vi "RichToFlatrfcontrol_DeviceStatusResponse.vi"(5 "OutputClusterType":T1, 11 "InputCluster":T2) -> (3 "OutputCluster":T1)   [LabVIEW 2024, in "FlexSDR_gRPC_client.lvlib"]
uses:
  rfcontrol_DeviceStatusResponse.ctl
  rfcontrol_DeviceStatusResponse_Flat.ctl
  FlexSDR_gRPC_client.lvlib
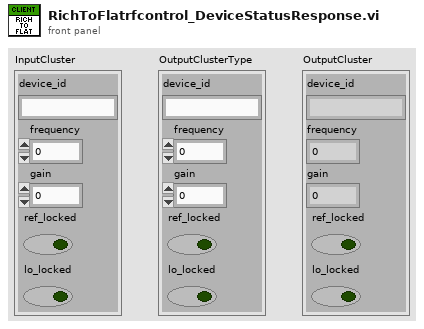
[diagram p1: front panel]
types:
  T1 = typedef "FlexSDR_gRPC_client.lvlib/rfcontrol_DeviceStatusResponse_Flat.ctl" = cluster{"device_id":string, "frequency":dbl, "gain":dbl, "ref_locked":bool, "lo_locked":bool}
  T2 = typedef "FlexSDR_gRPC_client.lvlib/rfcontrol_DeviceStatusResponse.ctl" = cluster{"device_id":string, "frequency":dbl, "gain":dbl, "ref_locked":bool, "lo_locked":bool}
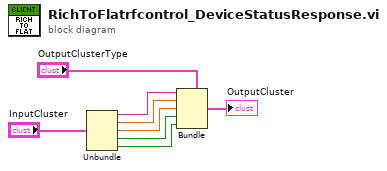
[diagram p0: block diagram]
diagram:
  n1 = Unbundle "Unbundle"("InputCluster") -> ("device_id"=w5:string, "frequency"=w4:dbl, "gain"=w3:dbl, "ref_locked"=w2:bool, "lo_locked"=w1:bool)
  n2 = Bundle "Bundle"(cluster="OutputClusterType", "device_id"=w5, "frequency"=w4, "gain"=w3, "ref_locked"=w2, "lo_locked"=w1) -> (→"OutputCluster":T1)
